vi "Send stop motors events.vi"(8 "error in (no error)":errorcluster, 9 "DAQ Module ID":i32, 10 "User Events":T1, 11 "Stop message":string) -> (0 "error out":errorcluster)   [LabVIEW 2020]
uses:
  controls/Motor direction ---typedef.ctl
  Controls/Motor controls---typedef.ctl
  controls/Continuous acquisition ---argument.ctl
  controls/Paused acquisition ---argument.ctl
  controls/Position arguments ---typedef.ctl
  controls/Move to zero ---argument.ctl
  controls/Timed acqn params ---typedef.ctl
  controls/User Events ---typedef.ctl
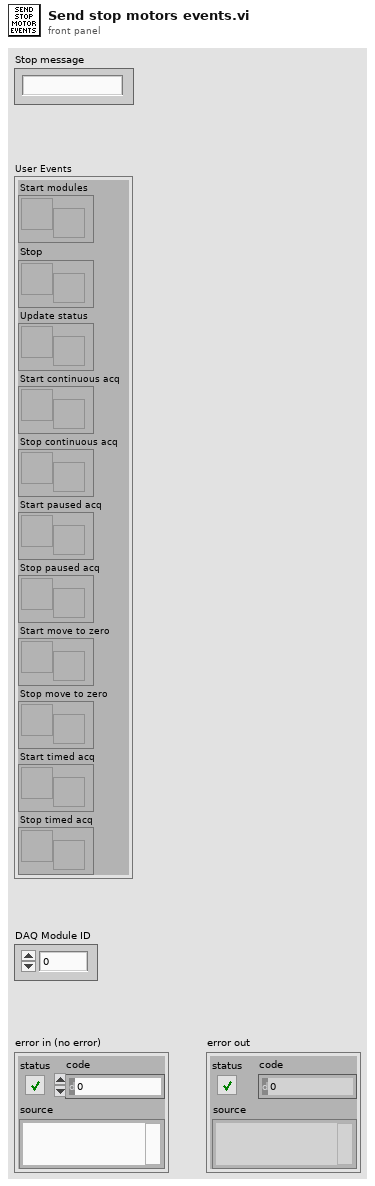
[diagram p1: front panel]
types:
  T1 = typedef "User Events ---typedef.ctl" = cluster{"Start modules":refnum<user-event>, "Stop":refnum<user-event>, "Update status":refnum<user-event>, "Start continuous acq":refnum<user-event>, "Stop continuous acq":refnum<user-event>, "Start paused acq":refnum<user-event>, "Stop paused acq":refnum<user-event>, "Start move to zero":refnum<user-event>, "Stop move to zero":refnum<user-event>, "Start timed acq":refnum<user-event>, "Stop timed acq":refnum<user-event>}
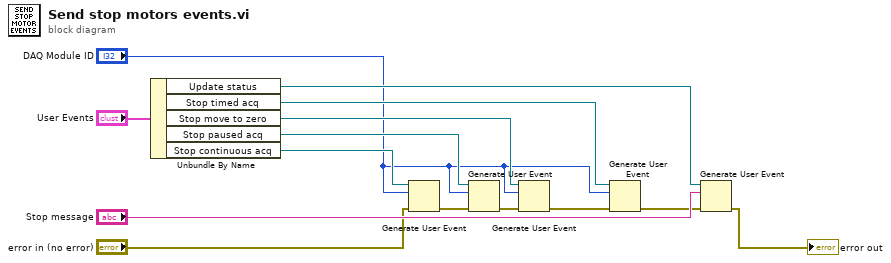
[diagram p0: block diagram]
diagram:
  n1 = Unbundle By Name("User Events") -> ("Update status"=w7:refnum<user-event>, "Stop timed acq"=w2:refnum<user-event>, "Stop move to zero"=w14:refnum<user-event>, "Stop paused acq"=w11:refnum<user-event>, "Stop continuous acq"=w8:refnum<user-event>)
  n2 = Generate User Event(user event=w8, event data cluster="DAQ Module ID", error in="error in (no error)") -> (error out=w10:errorcluster)  [unwired: 1 in, 1 out]
  n3 = Generate User Event(user event=w11, event data cluster="DAQ Module ID", error in=w10) -> (error out=w12:errorcluster)  [unwired: 1 in, 1 out]
  n4 = Generate User Event(user event=w14, event data cluster="DAQ Module ID", error in=w12) -> (error out=w13:errorcluster)  [unwired: 1 in, 1 out]
  n5 = Generate User Event(user event=w2, event data cluster="DAQ Module ID", error in=w13) -> (error out=w3:errorcluster)  [unwired: 1 in, 1 out]
  n6 = Generate User Event(user event=w7, event data cluster="Stop message", error in=w3) -> (error out=→"error out":errorcluster)  [unwired: 1 in, 1 out]
